vi "AddToMenu.vi"(8 "error in (no error)":errorcluster, 9 "ParentTag":string, 10 "MenuItem in":refnum<class "MGI_MenuItem.lvclass">, 11 "MGI_Menu in":refnum<class "MGI_Menu.lvclass">) -> (0 "error out":errorcluster, 2 "MenuItem out":refnum<class "MGI_MenuItem.lvclass">, 3 "MGI_Menu out":refnum<class "MGI_Menu.lvclass">)   [LabVIEW 2016, in "MGI_Menu.lvclass"]
doc: "Performs the actual add function on the menu.\n\nAuthored by Derek E. Trepanier\nsupport@mooregoodideas.com\nwww.mooregoodideas.com\n\nCopyright (c) 2012, Moore Good Ideas, Inc.\n\nAll rights reserved.\n\nRedistribution and use in source and binary forms, with or without modification, are permitted provided that the following conditions are met:\n\n * Redistributions of source code must retain the above copyright notice, this list of conditions and the following disclaimer.\n * Redistributions in binary form must reproduce the above copyright notice, this list of conditions and the following disclaimer in the documentation and/or other materials provided with the distribution.\n * Neither the name of Moore Good Ideas, Inc. nor the names of its contributors may be used to endorse or promote products derived from this software without specific prior written permission.\n\nTHIS SOFTWARE IS PROVIDED BY THE COPYRIGHT HOLDERS AND CONTRIBUTORS \"AS IS\" AND ANY EXPRESS OR IMPLIED WARRANTIES, INCLUDING, BUT NOT LIMITED TO, THE IMPLIED WARRANTIES OF MERCHANTABILITY AND FITNESS FOR A PARTICULAR PURPOSE ARE DISCLAIMED. IN NO EVENT SHALL THE COPYRIGHT OWNER OR CONTRIBUTORS BE LIABLE FOR ANY DIRECT, INDIRECT, INCIDENTAL, SPECIAL, EXEMPLARY, OR CONSEQUENTIAL DAMAGES (INCLUDING, BUT NOT LIMITED TO, PROCUREMENT OF SUBSTITUTE GOODS OR SERVICES; LOSS OF USE, DATA, OR PROFITS; OR BUSINESS INTERRUPTION) HOWEVER CAUSED AND ON ANY THEORY OF LIABILITY, WHETHER IN CONTRACT, STRICT LIABILITY, OR TORT (INCLUDING NEGLIGENCE OR OTHERWISE) ARISING IN ANY WAY OUT OF THE USE OF THIS SOFTWARE, EVEN IF ADVISED OF THE POSSIBILITY OF SUCH DAMAGE."
uses:
  <userlib>/_MGI/Menu Building/MenuTypes/MGI_Menu.lvclass
  <userlib>/_MGI/Menu Building/MenuItem/MGI_MenuItem.lvclass
  <userlib>/_MGI/Menu Building/MenuItem/Read Sub-Menus.vi
  <userlib>/_MGI/Menu Building/MenuItem/Read Full Tag.vi
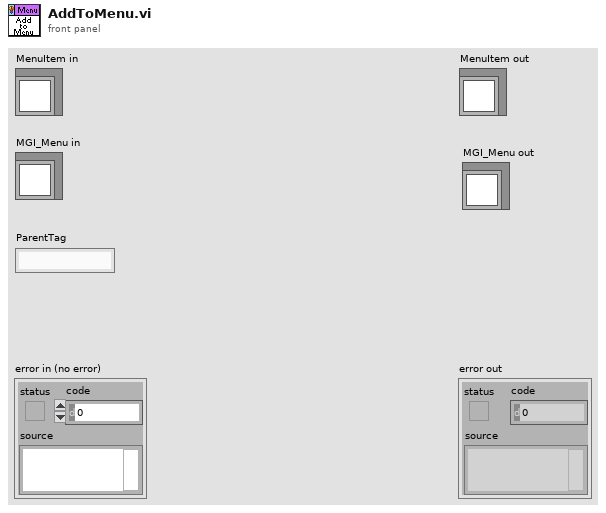
[diagram p1: front panel]
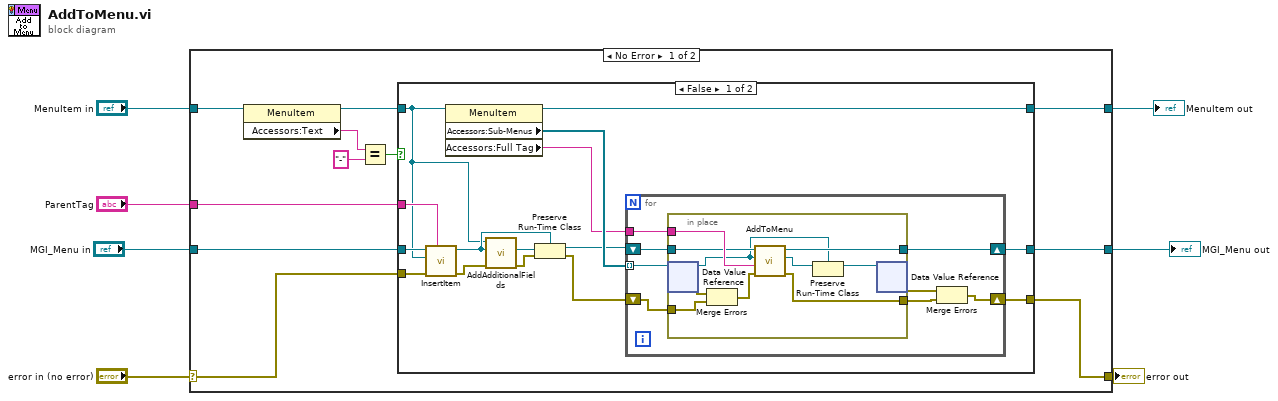
[diagram p0: block diagram]
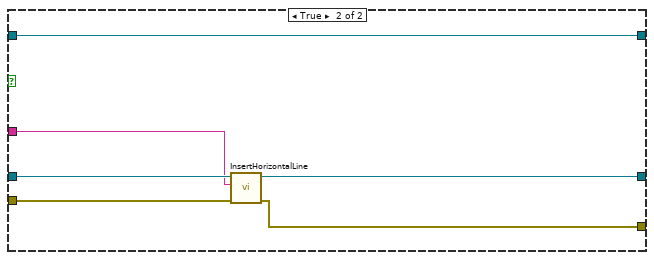
[diagram p2: hidden frame]
diagram:
  n1 = case shown="No Error" "error in (no error)" {
    selector: "error in (no error)" -> [w14 w60]
    tunnel: [w18 w60] -> w6
    tunnel: [w13 w59] -> w4
    tunnel: "MenuItem in" -> [w15 w59]
    tunnel: "MGI_Menu in" -> [w16 w58]
    tunnel: "ParentTag" -> [w17 _]
    tunnel: [w12 w58] -> w1
    frame No Error {
      n2 = property class="MenuItem"(reference=w15) -> (reference out=w10:refnum<class "MGI_MenuItem.lvclass">, "Accessors:Text"=w9:string)  [unwired: 1 in, 1 out]
      n3 = Equal?(x=w9, y="-") -> (x = y?=w8:bool)
      n4 = case shown="False" w8 {
        tunnel: [w32 w52] -> w18
        tunnel: w17 -> [w31 w56]
        tunnel: w16 -> [w29 w57]
        tunnel: w10 -> [w22 w54]
        tunnel: w14 -> [w28 w53]
        tunnel: [w27 w54] -> w13
        tunnel: [w26 w55] -> w12
        frame False {
          n5 = call-dynamic "InsertItem.vi"("Parent Tag"=w31, "error in (no error)"=w28, "MenuItem"=w22, "Menu in"=w29) -> ("error out"=w21:errorcluster, "Menu out"=w24:refnum<class "MGI_Menu.lvclass">)  [unwired: 6 in]
          n6 = property class="MenuItem"(reference=w22) -> (reference out=w27:refnum<class "MGI_MenuItem.lvclass">, "Accessors:Sub-Menus"=w33:refnum<data-value>[], "Accessors:Full Tag"=w30:string)  [unwired: 1 in, 1 out]
          n7 = call-dynamic "AddAdditionalFields.vi"("error in (no error)"=w21, "Menu"=w24, "MenuItem in"=w22) -> ("error out"=w20:errorcluster, "Menu out"=w25:refnum<class "MGI_Menu.lvclass">)  [unwired: 6 in, 1 out]
          n8 = Preserve Run-Time Class(object in=w25, error in=w20, 2:w24) -> (object out=w23:refnum<class "MGI_Menu.lvclass">, error out=w19:errorcluster)
          n9 = for {
            tunnel: w33 -> [w41] mode=indexing
            tunnel: w30 -> [w40]
            shift-right: [w38] -> w32
            shift-left: w19 -> [w36]
            shift-right: [w34] -> w26
            shift-left: w23 -> [w35]
            n10 = in-place {
              in-place-border: w40 -> [w51]
              in-place-border: [w50] -> w37
              in-place-border: w36 -> [w49]
              in-place-border: w35 -> [w46]
              in-place-border: [w45] -> w34
              n11 = in-place-dvr #1(w41) -> (w42:refnum<class "MGI_MenuItem.lvclass">, w48:errorcluster)
              n12 = Merge Errors(w48, w49) -> (w47:errorcluster)
              n13 = call-dynamic "AddToMenu.vi"("error in (no error)"=w47, "ParentTag"=w51, "MenuItem in"=w42, "MGI_Menu in"=w46) -> ("error out"=w50:errorcluster, "MenuItem out"=w44:refnum<class "MGI_MenuItem.lvclass">, "MGI_Menu out"=w45:refnum<class "MGI_Menu.lvclass">)  [unwired: 5 in]
              n14 = Preserve Run-Time Class(object in=w44, 2:w42) -> (object out=w43:refnum<class "MGI_MenuItem.lvclass">)  [unwired: 1 in, 1 out]
              n15 = in-place-dvr #1(w43) -> (w39:errorcluster)  [unwired: 1 out]
            }
            n16 = Merge Errors(w39, w37) -> (w38:errorcluster)
          }
        }
        frame True {
          n17 = call-dynamic "InsertHorizontalLine.vi"("error in (no error)"=w53, "ParentTag"=w56, "Menu in"=w57) -> ("error out"=w52:errorcluster, "Menu out"=w55:refnum<class "MGI_Menu.lvclass">)  [unwired: 7 in]
        }
      }
    }
    frame Error {
    }
  }
  "error out" <- w6
  "MenuItem out" <- w4
  "MGI_Menu out" <- w1
